vi "Do.vi"(8 "error in (no error)":errorcluster caption="错误输入（无错误）", 10 "Actor in":refnum<class "Actor.lvclass"> caption="操作者输入", 11 "框中控件消息":refnum<class "框中控件消息.lvclass">) -> (0 "error out":errorcluster caption="错误输出", 2 "Actor out":refnum<class "Actor.lvclass"> caption="操作者输出")   [LabVIEW 2018, in "程序响应.lvlib" / "框中控件消息.lvclass"]
doc: "本VI通过对操作者调用合适的方法，将消息发送给操作者。"
uses:
  <vilib>/ActorFramework/Actor/Actor.lvclass
  C:/Program Files (x86)/National Instruments/LabVIEW 2018/vi.lib/ActorFramework/Actor/Actor.lvclass
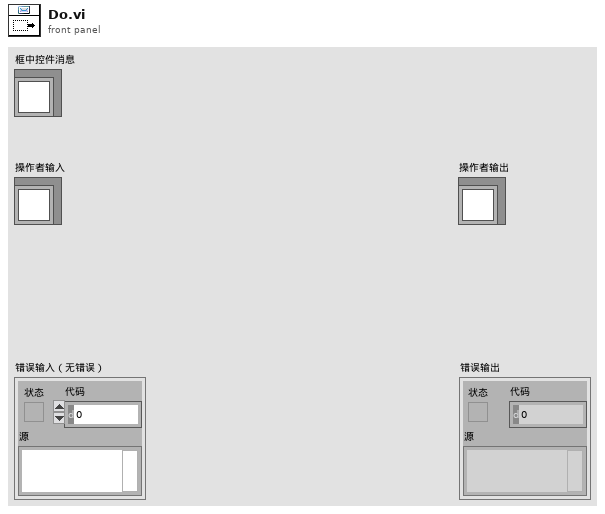
[diagram p1: front panel]
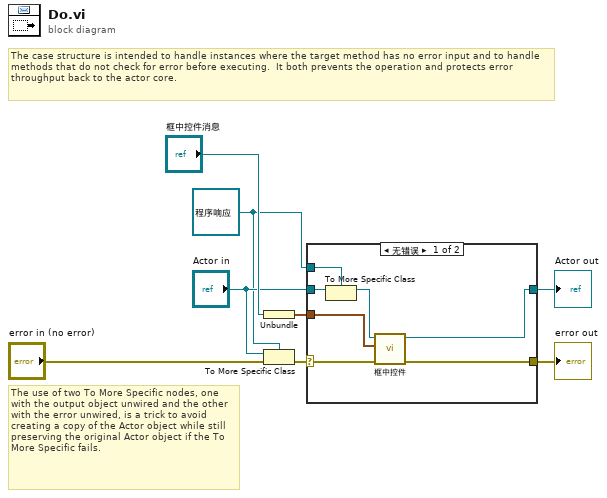
[diagram p0: block diagram]
diagram:
  w2 = refnum<class "程序响应.lvclass"> refnum ("Actor in")
  # "The use of two To More Specific nodes, one with the output object unwired and the other with the error unwired, is a trick to avoid creating a copy of the Actor object while still preserving the original Actor object if the To More Specific fails."
  # "The case structure is intended to handle instances where the target method has no error input and to handle methods that do not check for error before executing.  It both prevents the operation and protects error throughput back to the actor core."
  n1 = Unbundle("框中控件消息") -> (w1:cluster{"Horizontal":i32, "Vertical":i32})
  n2 = To More Specific Class(target class=w2, reference="Actor in", error in="error in (no error)") -> (error out=w6:errorcluster)  [unwired: 1 out]
  n3 = case shown="无错误" w6 {
    selector: w6 -> [w13 w17]
    tunnel: [w15 w17] -> w5
    tunnel: [w14 w16] -> w4
    tunnel: "Actor in" -> [w12 w16]
    tunnel: w2 -> [w11 _]
    tunnel: w1 -> [w9 _]
    frame No Error {
      n4 = To More Specific Class(target class=w11, reference=w12) -> (specific class reference=w10:refnum<class "程序响应.lvclass">)  [unwired: 1 in, 1 out]
      n5 = call-dynamic "框中控件.vi"("error in (no error)"=w13, "结束坐标"=w9, "程序响应 输入"=w10) -> ("error out"=w15:errorcluster, "程序响应 输出"=w14:refnum<class "程序响应.lvclass">)  [unwired: 7 in]
    }
    frame Error {
      # "If type check fails, pass the original object out again."
    }
  }
  "error out" <- w5
  "Actor out" <- w4
